vi "SRV_Evaluate Formula.vi"() -> ()   [LabVIEW 2014]
doc: "Evaluates the input formulas.\n\n\nAuthor: Mike Schultz - Logic PD"
uses:
  <vilib>/gmath/NI_Gmath.lvlib
panel:
  in  "error in (no error)":errorcluster
  out "error out":errorcluster
  out "Output Values":dbl[](array[numeric])
  in  "Variables Input":string[](array[string])=["r", "p"]
  in  "formulas":string="d = 2 * r ; \na = p * r ^ 2 ; \nc = 2 * p * r"
  in  "Input Values":dbl[](array[numeric])=[5.0, 3.1415]
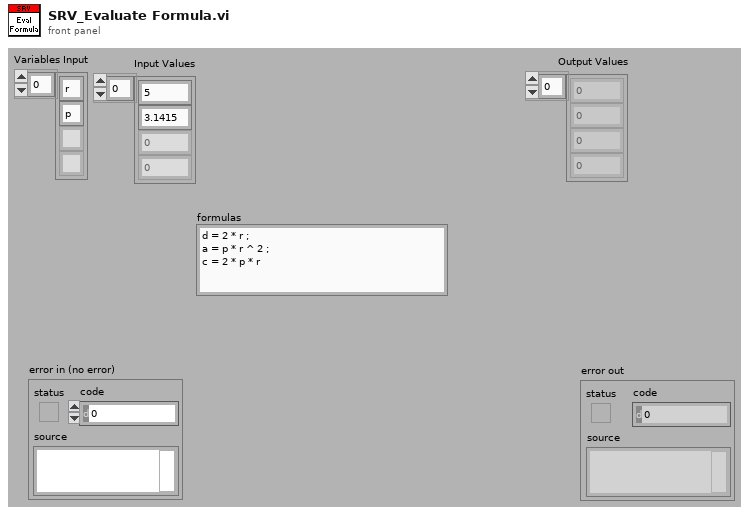
[diagram p1: front panel]
types:
  T1 = cluster{"Y Values":dbl[][], "Tables":i32[][][], "Variables input decode":i32[], "Variables output decode":i32[]}
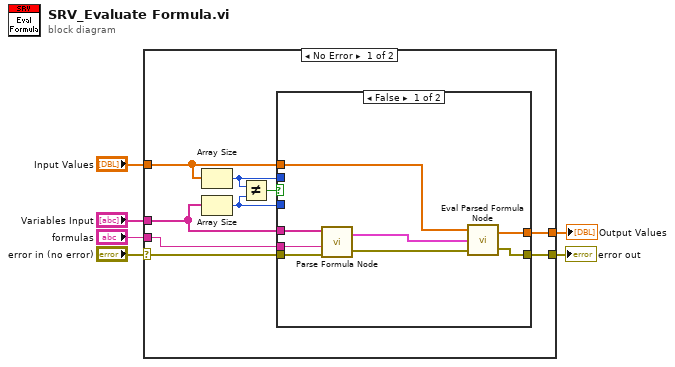
[diagram p0: block diagram]
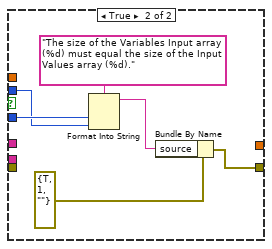
[diagram p2: hidden frame]
diagram:
  n1 = case shown="No Error" "error in (no error)" {
    selector: "error in (no error)" -> [w7 w30]
    tunnel: [w15 _] -> w6
    tunnel: "formulas" -> [w14 _]
    tunnel: [w13 w30] -> w4
    tunnel: "Input Values" -> [w12 _]
    tunnel: "Variables Input" -> [w11 _]
    frame No Error {
      n2 = Array Size(array=w12) -> (size(s)=w9:i32)
      n3 = Array Size(array=w11) -> (size(s)=w8:i32)
      n4 = Not Equal?(x=w9, y=w8) -> (x != y?=w10:bool)
      n5 = case shown="False" w10 {
        tunnel: [w23 _] -> w15
        tunnel: w14 -> [w21 _]
        tunnel: [w19 w25] -> w13
        tunnel: w7 -> [w18 _]
        tunnel: w12 -> [w17 _]
        tunnel: w11 -> [w16 _]
        tunnel: w9 -> [_ w27]
        tunnel: w8 -> [_ w28]
        frame False {
          n6 = call <vilib>:"Parse Formula Node.vi"("error in (no error)"=w18, "formula"=w21, "Variables Input"=w16) -> ("error out"=w22:errorcluster, "Parsed Formula Node"=w20:T1)  [unwired: 1 in]
          n7 = call <vilib>:"Eval Parsed Formula Node.vi"("error in (no error)"=w22, "Parsed Formula Node"=w20, "Input Values"=w17) -> ("error out"=w19:errorcluster, "Output Values"=w23:dbl[])
        }
        frame True {
          n8 = Format Into String(format string="The size of the Variables Input array (%d) must equal the size of the Input Values array (%d).", w28, w27) -> (resulting string=w24:string)  [unwired: 2 in, 1 out]
          n9 = Bundle By Name(cluster=errorcluster {"status"=TRUE, "code"=1, "source"=""} ("error out"), "source"=w24) -> (w25:errorcluster)
        }
      }
    }
    frame Error {
    }
  }
  "Output Values" <- w6
  "error out" <- w4
